vi "Write Base Actor.vi"(10 "Base Actor":T1, 11 "Base Actor in":refnum<class "Base Actor.lvclass">) -> (3 "Base Actor out":refnum<class "Base Actor.lvclass">)   [LabVIEW 2020, in "jettl.lvlib" / "Base jettl Actor.lvlib" / "Base Actor.lvlib" / "Base Actor.lvclass"]
uses:
  Base Actor.lvclass
  Base Actor.lvclass/Base Actor.ctl
  Unified Actor Lifetime.ctl
  jettl.lvlib
  Base Actor.ctl
  Msg Input/Msg Input.lvclass
  Msg Output/Msg Output.lvclass
  Msg/Msg.lvclass
  Unified Actor Relation.ctl
  Teller.ctl
  Msg.ctl
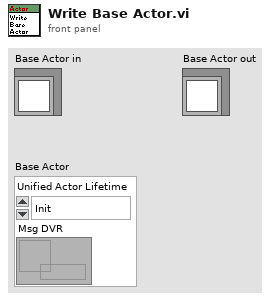
[diagram p1: front panel]
types:
  T1 = typedef "jettl.lvlib/Base Actor.ctl" = cluster{"Unified Actor Lifetime":T2, "Msg DVR":refnum<data-value>}
  T2 = typedef "jettl.lvlib/Unified Actor Lifetime.ctl" = enum16{"Init", "Spawn", "Setup", "Teardown Before Running", "Running", "Stop Called", "Stopping With Children", "Stopping Without Children", "Teardown After Running", "Stopped"}
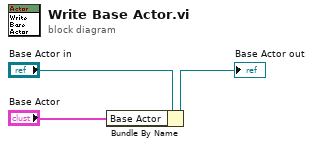
[diagram p0: block diagram]
diagram:
  n1 = Bundle By Name(cluster="Base Actor in", "Base Actor"="Base Actor") -> (→"Base Actor out":refnum<class "Base Actor.lvclass">)
